vi "Cleanup.vi"(8 "error in (no error)":errorcluster, 11 "Mixer in":refnum<class "Transport.lvclass">) -> (0 "error out":errorcluster)   [LabVIEW 2020, in "Transport.lvclass"]
uses:
  Transport.lvclass
  Transport.lvclass/Transport.ctl
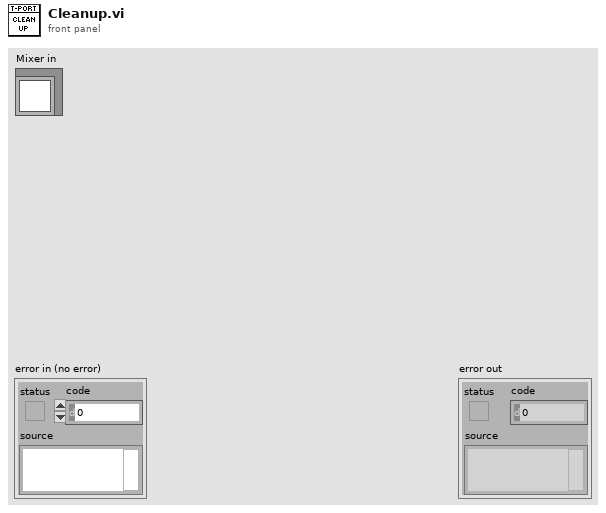
[diagram p1: front panel]
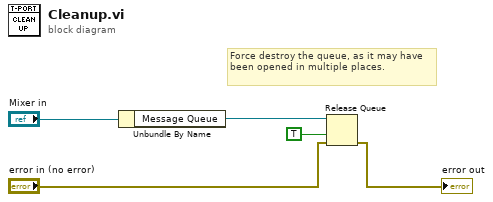
[diagram p0: block diagram]
diagram:
  # "Force destroy the queue, as it may have been opened in multiple places."
  n1 = Unbundle By Name("Mixer in") -> ("Message Queue"=w2:refnum<queue>)
  n2 = Release Queue(queue=w2, force destroy? (F)=TRUE, error in (no error)="error in (no error)") -> (error out=→"error out":errorcluster)  [unwired: 2 out]
